vi "Downable_i.vi"(1 "背景":dbl[][](array[numeric]), 2 "方块":dbl[][](array[numeric]), 3 "point":cluster{"x":i16, "y":i16} caption="位置") -> (0 "输出":bool)   [LabVIEW 2016]
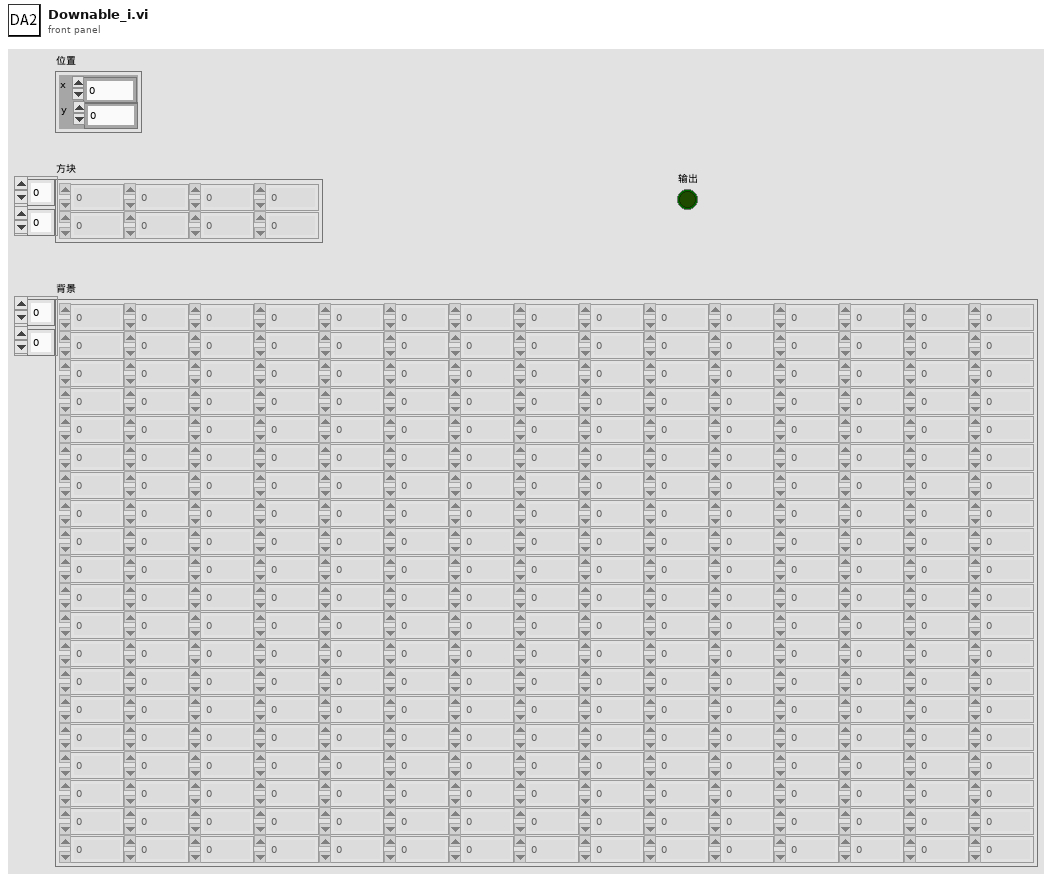
[diagram p1: front panel]
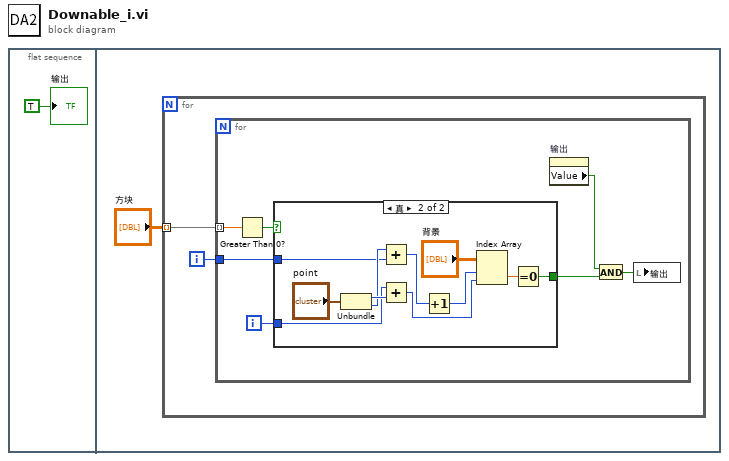
[diagram p0: block diagram]
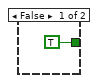
[diagram p2: hidden frame]
diagram:
  n1 = flat-sequence {
    frame #0 {
      "输出" <- TRUE
    }
    frame #1 {
      n2 = for {
        tunnel: "方块" -> [w4] mode=indexing
        i -> [w3]
        n3 = for {
          tunnel: w4 -> [w11] mode=indexing
          tunnel: w3 -> [w8]
          i -> [w9]
          n4 = Greater Than 0?(x=w11) -> (x > 0?=w10:bool)
          n5 = case shown="真" w10 {
            tunnel: w9 -> [_ w22]
            tunnel: w8 -> [_ w20]
            tunnel: [TRUE w14] -> w7
            frame False {
            }
            frame True {
              n6 = Unbundle("point") -> ("x"=w23:i16, "y"=w21:i16)
              n7 = Add(x=w21, y=w20) -> (x+y=w19:i32)
              n8 = Add(x=w22, y=w23) -> (x+y=w17:i32)
              n9 = Increment(x=w19) -> (x+1=w16:i32)
              n10 = Index Array(array="背景", index (row)=w16, index (col)=w17) -> (element=w15:dbl)
              n11 = Equal To 0?(x=w15) -> (x = 0?=w14:bool)
            }
          }
          n12 = property on="输出" class="Bool (严格)"() -> ("Value"=w6:bool)  [unwired: 2 in, 2 out]
          n13 = And(x=w6, y=w7) -> (x .and. y?=w5:bool)
          n14 = local write "输出"(w5) -> ()
        }
      }
    }
  }
